vi "HEALTH_LABVIEW_V5.vi"() -> ()   [LabVIEW 2026]
uses:
  <vilib>/addons/control/pid/pid.llb/PID (DBL).vi
  <vilib>/addons/control/pid/NI_PID_pid.lvlib
panel:
  out "Value":dbl format="%.2f"
  in  "CLEAR GRAPHS":bool
  in  "TEMP SENSOR\nZEROING VALUE (C)":dbl
  in  "FLOW PID gains":T1={"proportional gain (Kc)"=1.0, "integral time (Ti, min)"=0.01, "derivative time (Td, min)"=0.0} {"derivative time (Td, min)" format="%.3f"; "integral time (Ti, min)" format="%.3f"; "proportional gain (Kc)" format="%.3f"}
  in  "TARGET FLOW RATE (LPM)":dbl format="%.2f"
  in  "HEATER PID gains":T1={"proportional gain (Kc)"=1.0, "integral time (Ti, min)"=0.01, "derivative time (Td, min)"=0.0} {"derivative time (Td, min)" format="%.3f"; "integral time (Ti, min)" format="%.3f"; "proportional gain (Kc)" format="%.3f"}
  out "HEATER SIDE BLOCK RTD":dbl(graph)
  out "OUTLET TEMP (C)":dbl format="%#_3g"
  out "INLET TEMP (C)":dbl format="%#_3g"
  out "INLET PRESSURE (PSI)":dbl(graph)
  out "PRESSURE DROP (PSI)":dbl(graph)
  out "DELTA T (C)":dbl format="%#_3f"
  out "DELTA T (C)":dbl(graph)
  out "COOLANT FLOW RATE":dbl(graph)
  in  "PUMP ON/OFF":bool
  out "HX SIDE BLOCK RTD":cluster{dbl, "TARGET HX TEMP (C)":dbl}(graph)
  out "HEATER POWER OUTPUT":dbl(knob) scale=0.0..100.0
  in  "TARGET HX TEMP (C)":dbl
  in  "HEATER ON/OFF":bool
  in  "stop":bool
  out "Error String":string
  out "error out":errorcluster
  out "ConnectionType Out":i32
  out "DeviceType Out":i32
  in  "Identifier":string="LJM_idANY"
  in  "ConnectionType":string="LJM_ctANY"
  in  "DeviceType":string="LJM_dtANY"
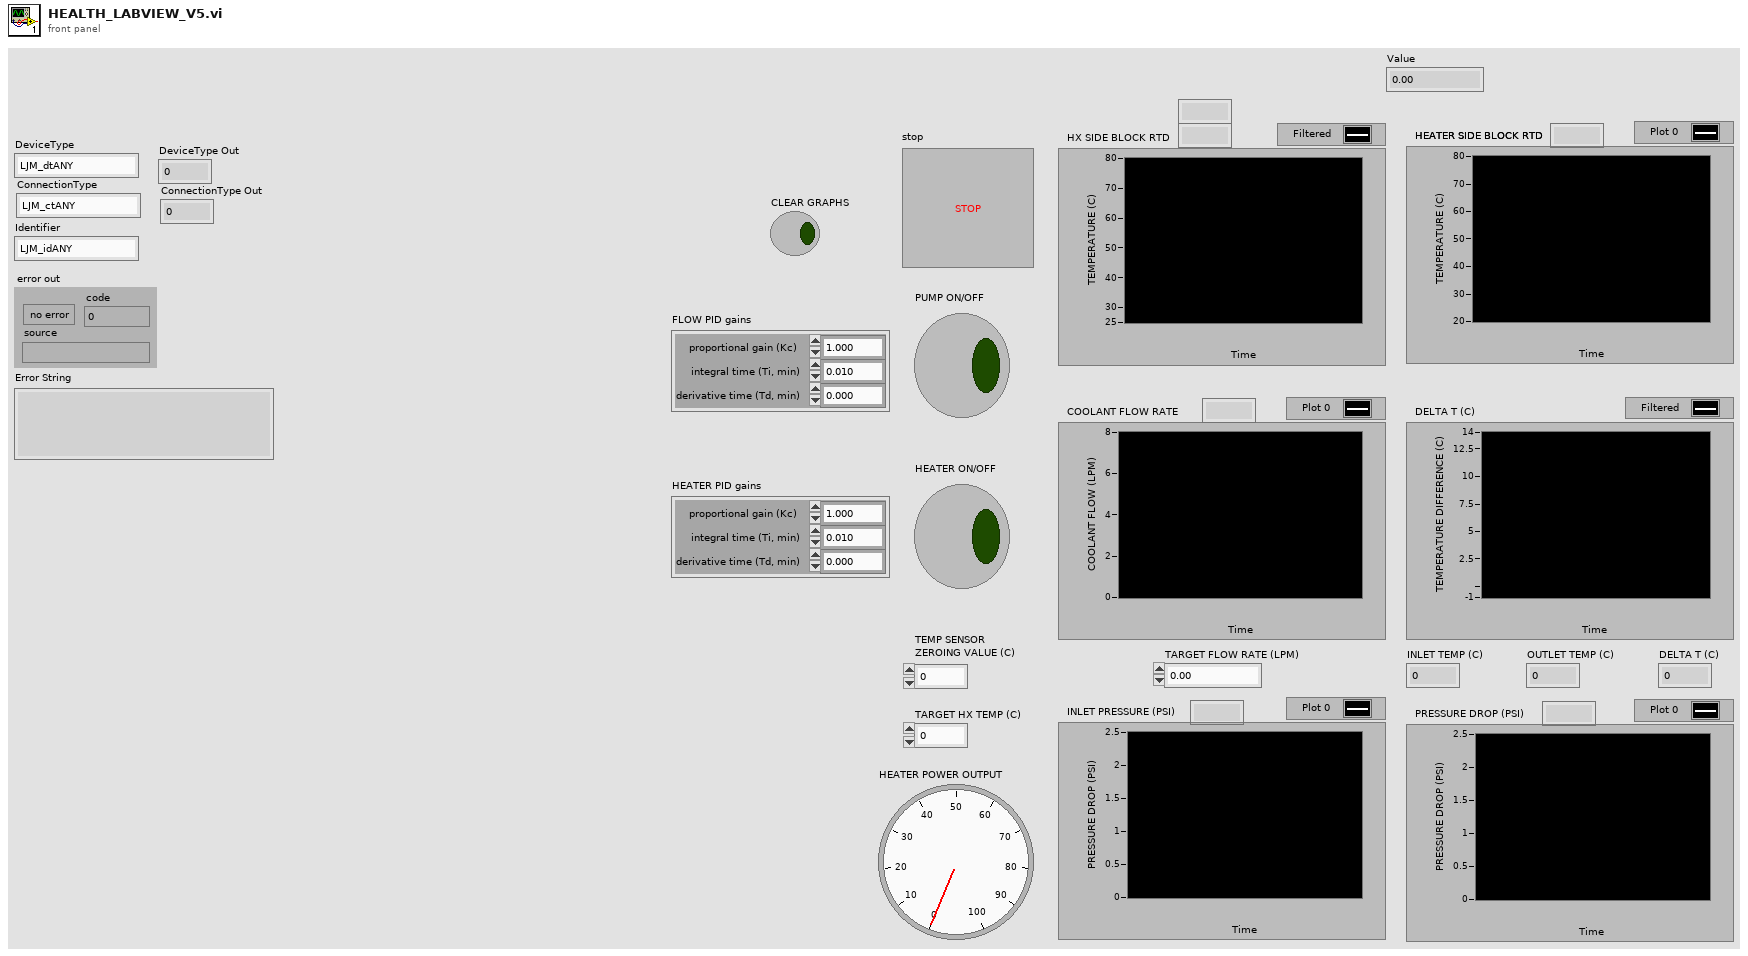
[diagram p1: front panel]
types:
  T1 = cluster{"proportional gain (Kc)":dbl, "integral time (Ti, min)":dbl, "derivative time (Td, min)":dbl}
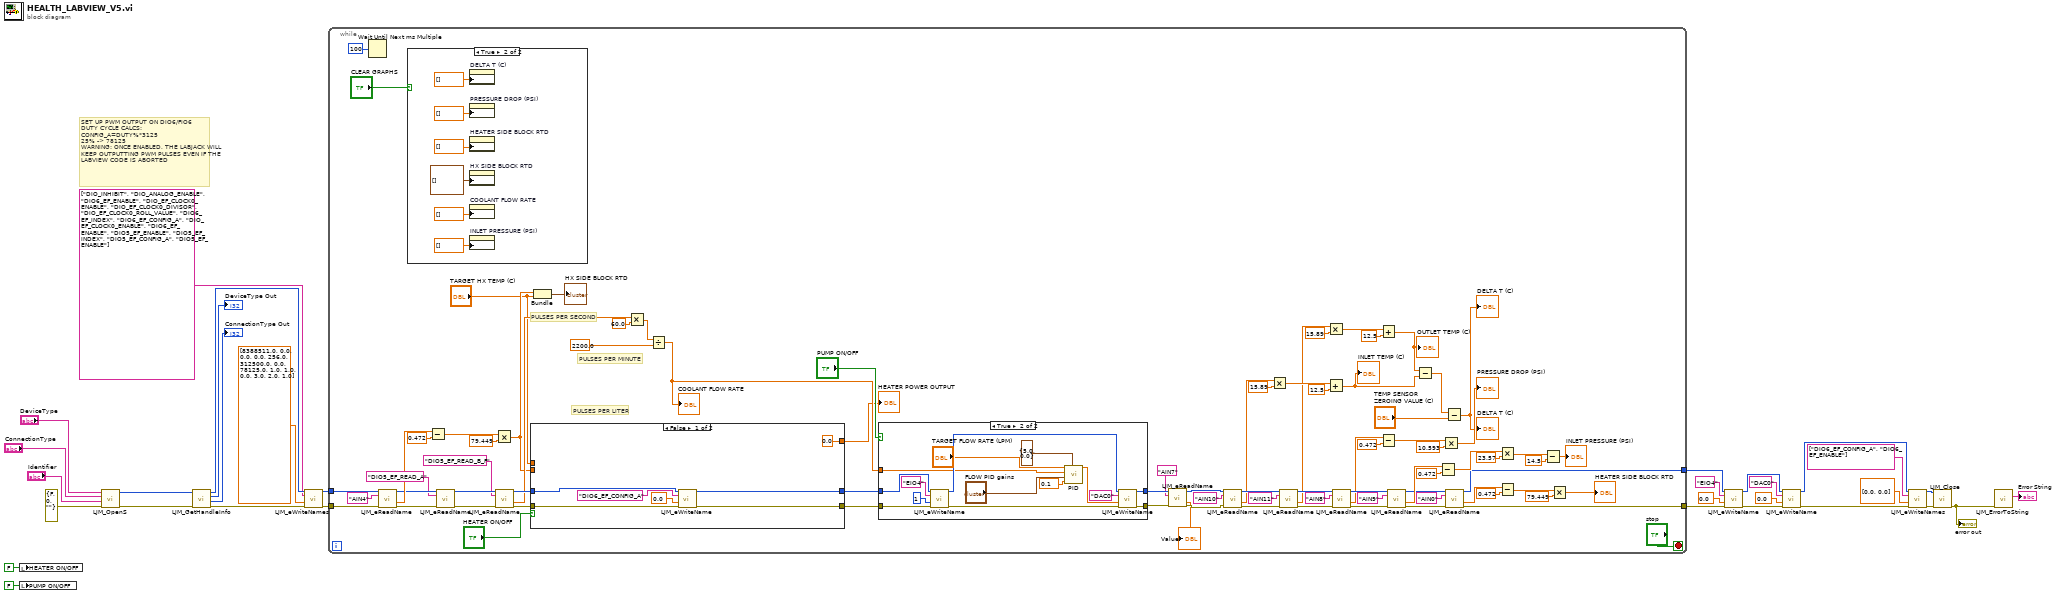
[diagram p0: block diagram]
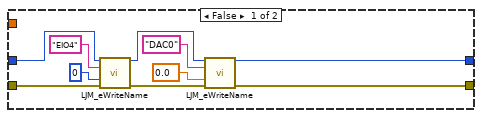
[diagram p3: hidden frame]
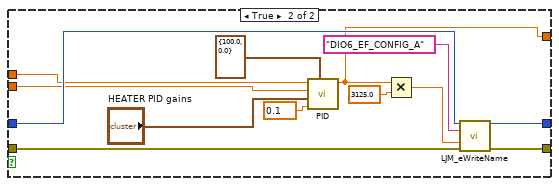
[diagram p4: hidden frame]
diagram:
  # "SET UP PWM OUTPUT ON DIO6/FIO6\nDUTY CYCLE CALCS:\nCONFIG_A=DUTY%*3125\n25% -> 78125\nWARNING: ONCE ENABLED, THE LABJACK WILL KEEP OUTPUTTING PWM PULSES EVEN IF THE LABVIEW CODE IS ABORTED"
  n1 = local write "HEATER ON/OFF"(FALSE ("HEATER ON/OFF 2")) -> ()
  n2 = local write "PUMP ON/OFF"(FALSE ("PUMP ON/OFF 2")) -> ()
  n3 = call "LJM_OpenS.vi"("error in"=errorcluster {"status"=FALSE, "code"=0, "source"=""} ("error in (no error)"), "Identifier"="Identifier", "ConnectionType"="ConnectionType", "DeviceType"="DeviceType") -> ("error out"=w31:errorcluster, "Handle"=w30:i32)  [unwired: 6 in]
  n4 = call "LJM_GetHandleInfo.vi"("error in"=w31, "Handle In"=w30) -> ("error out"=w21:errorcluster, "ConnectionType"=→"ConnectionType Out":i32, "DeviceType"=→"DeviceType Out":i32, "Handle Out"=w22:i32)  [unwired: 2 in, 4 out]
  n5 = call "LJM_eWriteNames.vi"("Handle In"=w22, "aNames"=string[] ["DIO_INHIBIT", "DIO_ANALOG_ENABLE", "DIO6_EF_ENABLE", "DIO_EF_CLOCK0_ENABLE", "DIO_EF_CLOCK0_DIVISOR", "DIO_EF_CLOCK0_ROLL_VALUE", "DIO6_EF_INDEX", "DIO6_EF_CONFIG_A", "DIO_EF_CLOCK0_ENABLE", "DIO6_EF_ENABLE", "DIO5_EF_ENABLE", "DIO5_EF_INDEX", "DIO5_EF_CONFIG_A", "DIO5_EF_ENABLE"], "aValuesIn"=dbl[] [8388511.0, 0.0, 0.0, 0.0, 256.0, 312500.0, 0.0, 78125.0, 1.0, 1.0, 0.0, 3.0, 2.0, 1.0], "error in"=w21) -> ("Handle Out"=w2:i32, "error out"=w1:errorcluster)  [unwired: 9 in, 1 out]
  n6 = while {
    tunnel: [w63] -> w9
    tunnel: w2 -> [w104]
    tunnel: w1 -> [w103]
    tunnel: [w64] -> w3
    stop <- "stop" stop-if-true
    # "PULSES PER LITER"
    # "PULSES PER MINUTE"
    # "PULSES PER SECOND"
    n7 = Wait Until Next ms Multiple(millisecond multiple=u32 100 ("milliseconds to wait")) -> ()  [unwired: 1 out]
    n8 = call "LJM_eReadName.vi"("Handle In"=w104, "Name"="AIN4", "error in"=w103) -> ("Handle Out"=w102:i32, "Value"=w110:dbl, "error out"=w101:errorcluster)  [unwired: 10 in]
    n9 = case shown="True" "CLEAR GRAPHS" {
      frame False {
      }
      frame True {
        n10 = property on="DELTA T (C)" class="WFChart (strict)"("History Data"=dbl[] []) -> ()  [unwired: 2 in, 2 out]
        n11 = property on="PRESSURE DROP (PSI)" class="WFChart (strict)"("History Data"=dbl[] []) -> ()  [unwired: 2 in, 2 out]
        n12 = property on="HEATER SIDE BLOCK RTD" class="WFChart (strict)"("History Data"=dbl[] []) -> ()  [unwired: 2 in, 2 out]
        n13 = property on="HX SIDE BLOCK RTD" class="WFChart (strict)"("History Data"=cluster{dbl, "TARGET HX TEMP (C)":dbl}[] []) -> ()  [unwired: 2 in, 2 out]
        n14 = property on="COOLANT FLOW RATE" class="WFChart (strict)"("History Data"=dbl[] []) -> ()  [unwired: 2 in, 2 out]
        n15 = property on="INLET PRESSURE (PSI)" class="WFChart (strict)"("History Data"=dbl[] []) -> ()  [unwired: 2 in, 2 out]
      }
    }
    n16 = Subtract(x=w110, y=0.472 ("Address 2")) -> (x-y=w113:dbl)
    n17 = call "LJM_eReadName.vi"("Handle In"=w102, "Name"="DIO5_EF_READ_A", "error in"=w101) -> ("Handle Out"=w99:i32, "error out"=w96:errorcluster)  [unwired: 10 in, 1 out]
    n18 = Multiply(x=w113, y=79.449 ("Address 2")) -> (x*y=w42:dbl)
    n19 = call "LJM_eReadName.vi"("Handle In"=w99, "Name"="DIO5_EF_READ_B_F" ("DIO5_EF_READ_B_F"), "error in"=w96) -> ("Handle Out"=w98:i32, "Value"=w57:dbl, "error out"=w97:errorcluster)  [unwired: 10 in]
    n20 = case shown="False" "HEATER ON/OFF" {
      tunnel: [w151 w165] -> w105
      tunnel: [w152 w164] -> w106
      tunnel: "TARGET HX TEMP (C)" -> [_ w157]
      tunnel: w42 -> [_ w158]
      tunnel: w98 -> [w148 w160]
      tunnel: w97 -> [w147 w159]
      tunnel: [0.0 ("output") w153] -> w40
      frame False {
        n21 = call "LJM_eWriteName.vi"("Handle In"=w148, "Name"="DIO6_EF_CONFIG_A", "Value"=0.0, "error in"=w147) -> ("Handle Out"=w152:i32, "error out"=w151:errorcluster)  [unwired: 10 in]
      }
      frame True {
        n22 = call-poly <vilib>:"PID.vi"("output range"=cluster{"output high":dbl, "output low":dbl} {"output high"=100.0, "output low"=0.0}, "dt (s)"=0.1, "PID gains"="HEATER PID gains", "process variable"=w158, "setpoint"=w157) -> ("output"=w153:dbl)  [unwired: 5 in, 1 out]
        n23 = Multiply(x=w153, y=3125.0) -> (x*y=w162:dbl)
        n24 = call "LJM_eWriteName.vi"("Handle In"=w160, "Name"="DIO6_EF_CONFIG_A", "Value"=w162, "error in"=w159) -> ("Handle Out"=w164:i32, "error out"=w165:errorcluster)  [unwired: 10 in]
      }
    }
    "HEATER POWER OUTPUT" <- w40
    n25 = Bundle(w42, "TARGET HX TEMP (C)"="TARGET HX TEMP (C)") -> (→"HX SIDE BLOCK RTD":cluster{dbl, "TARGET HX TEMP (C)":dbl})  [unwired: 1 in]
    n26 = Multiply(x=w57, y=60.0) -> (x*y=w55:dbl)
    n27 = Divide(x=w55, y=2200.0) -> (x/y=w53:dbl)
    "COOLANT FLOW RATE" <- w53
    n28 = case shown="True" "PUMP ON/OFF" {
      tunnel: w106 -> [w128 w143]
      tunnel: w105 -> [w127 w142]
      tunnel: [w123 w137] -> w36
      tunnel: [w122 w138] -> w35
      tunnel: w53 -> [_ w136]
      frame False {
        n29 = call "LJM_eWriteName.vi"("Handle In"=w128, "Name"="EIO4", "Value"=0, "error in"=w127) -> ("Handle Out"=w125:i32, "error out"=w124:errorcluster)  [unwired: 10 in]
        n30 = call "LJM_eWriteName.vi"("Handle In"=w125, "Name"="DAC0", "Value"=0.0, "error in"=w124) -> ("Handle Out"=w122:i32, "error out"=w123:errorcluster)  [unwired: 10 in]
      }
      frame True {
        n31 = call "LJM_eWriteName.vi"("Handle In"=w143, "Name"="EIO4", "Value"=1, "error in"=w142) -> ("Handle Out"=w139:i32, "error out"=w140:errorcluster)  [unwired: 10 in]
        n32 = call-poly <vilib>:"PID.vi"("output range"=cluster{"output high":dbl, "output low":dbl} {"output high"=5.0, "output low"=0.0}, "dt (s)"=0.1 ("FLOW dt (s)"), "PID gains"="FLOW PID gains", "process variable"=w136, "setpoint"="TARGET FLOW RATE (LPM)") -> ("output"=w131:dbl)  [unwired: 5 in, 1 out]
        n33 = call "LJM_eWriteName.vi"("Handle In"=w139, "Name"="DAC0", "Value"=w131, "error in"=w140) -> ("Handle Out"=w138:i32, "error out"=w137:errorcluster)  [unwired: 10 in]
      }
    }
    n34 = call "LJM_eReadName.vi"("Handle In"=w35, "Name"="AIN7", "error in"=w36) -> ("Handle Out"=w38:i32, "Value"=→"Value":dbl, "error out"=w37:errorcluster)  [unwired: 10 in]
    n35 = call "LJM_eReadName.vi"("Handle In"=w38, "Name"="AIN10", "error in"=w37) -> ("Handle Out"=w94:i32, "Value"=w51:dbl, "error out"=w91:errorcluster)  [unwired: 10 in]
    n36 = Multiply(x=w51, y=15.89) -> (x*y=w83:dbl)
    n37 = call "LJM_eReadName.vi"("Handle In"=w94, "Name"="AIN11" ("Name 2"), "error in"=w91) -> ("Handle Out"=w93:i32, "Value"=w50:dbl, "error out"=w90:errorcluster)  [unwired: 10 in]
    n38 = Multiply(x=w50, y=15.89) -> (x*y=w80:dbl)
    n39 = Add(x=w83, y=12.5) -> (x+y=w48:dbl)
    "INLET TEMP (C)" <- w48
    n40 = call "LJM_eReadName.vi"("Handle In"=w93, "Name"="AIN8" ("Name 3"), "error in"=w90) -> ("Handle Out"=w92:i32, "Value"=w67:dbl, "error out"=w89:errorcluster)  [unwired: 10 in]
    n41 = Add(x=w80, y=12.5) -> (x+y=w49:dbl)
    "OUTLET TEMP (C)" <- w49
    n42 = Subtract(x=w67, y=0.472) -> (x-y=w77:dbl)
    n43 = call "LJM_eReadName.vi"("Handle In"=w92, "Name"="AIN9" ("Name 4"), "error in"=w89) -> ("Handle Out"=w66:i32, "Value"=w71:dbl, "error out"=w65:errorcluster)  [unwired: 10 in]
    n44 = Subtract(x=w49, y=w48) -> (x-y=w47:dbl)
    n45 = Subtract(x=w71, y=0.472) -> (x-y=w73:dbl)
    n46 = Multiply(x=w77, y=10.593) -> (x*y=→"PRESSURE DROP (PSI)":dbl)
    n47 = Subtract(x=w47, y="TEMP SENSOR\nZEROING VALUE (C)") -> (x-y=→"DELTA T (C)" →"DELTA T (C)":dbl)
    n48 = call "LJM_eReadName.vi"("Handle In"=w66, "Name"="AIN0", "error in"=w65) -> ("Handle Out"=w63:i32, "Value"=w58:dbl, "error out"=w64:errorcluster)  [unwired: 10 in]
    n49 = Multiply(x=w73, y=23.57) -> (x*y=w69:dbl)
    n50 = Subtract(x=w58, y=0.472 ("Address 2")) -> (x-y=w61:dbl)
    n51 = Subtract(x=w69, y=14.5) -> (x-y=→"INLET PRESSURE (PSI)":dbl)
    n52 = Multiply(x=w61, y=79.449 ("Address 2")) -> (x*y=→"HEATER SIDE BLOCK RTD":dbl)
  }
  n53 = call "LJM_eWriteName.vi"("Handle In"=w9, "Name"="EIO4", "Value"=0.0, "error in"=w3) -> ("Handle Out"=w10:i32, "error out"=w13:errorcluster)  [unwired: 10 in]
  n54 = call "LJM_eWriteName.vi"("Handle In"=w10, "Name"="DAC0", "Value"=0.0, "error in"=w13) -> ("Handle Out"=w11:i32, "error out"=w12:errorcluster)  [unwired: 10 in]
  n55 = call "LJM_eWriteNames.vi"("Handle In"=w11, "aNames"=string[] ["DIO6_EF_CONFIG_A", "DIO6_EF_ENABLE"], "aValuesIn"=dbl[] [0.0, 0.0], "error in"=w12) -> ("Handle Out"=w17:i32, "error out"=w18:errorcluster)  [unwired: 9 in, 1 out]
  n56 = call "LJM_Close.vi"("error in"=w18, "Handle"=w17) -> ("error out"=w23:errorcluster)  [unwired: 9 in]
  "error out" <- w23
  n57 = call "LJM_ErrorToString.vi"("error in"=w23) -> ("String"=→"Error String":string)  [unwired: 10 in]
